vi "1_Sin(x)_Cos(x)(Training).vi"() -> ()   [LabVIEW 2020]
uses:
  <vilib>/Ngene/DeepLTK/Toolkit/NN_Train/Controls/NN_Train_Params.ctl
  <vilib>/Ngene/DeepLTK/Toolkit/NN_Train/Controls/NN_Train_Optimizer.ctl
  <vilib>/Ngene/DeepLTK/Toolkit/NN_Train/Controls/NN_Train_Data_Sampling.ctl
  <vilib>/Ngene/DeepLTK/Toolkit/NN_Train/Controls/NN_LR_Policy_Cfg.ctl
  <vilib>/Ngene/DeepLTK/Toolkit/NN_Train/Controls/NN_LR_Policy_Type.ctl
  <vilib>/Ngene/DeepLTK/Toolkit/NN_Train/Controls/NN_Train_Session_Data.ctl
  <vilib>/Ngene/DeepLTK/Toolkit/NN_Layers/Layers/FC/Controls/NN_Layer_Config(FC).ctl
  <vilib>/Ngene/DeepLTK/Toolkit/NN_Activations/Controls/NN_Activation_Type.ctl
  <vilib>/Ngene/DeepLTK/Toolkit/NN_Layers/Controls/NN_Layer_Init_Params.ctl
  <vilib>/Ngene/DeepLTK/Toolkit/NN_Layers/Controls/NN_Layer_Weight_Init_Type.ctl
  <vilib>/Ngene/DeepLTK/Toolkit/NN_Network/Controls/NN_Save_Before_Destroy_Options.ctl
  <vilib>/Ngene/DeepLTK/Toolkit/NN_Network/Controls/NN_Device.ctl
  <vilib>/Ngene/DeepLTK/Toolkit/NN_Layers/Layers/Input/Controls/NN_Layer_Config(Input1D).ctl
  <vilib>/Ngene/DeepLTK/Toolkit/NN_Data/API/DataSet_Types/NN_DataSet(In1D_Out1D).ctl
  <vilib>/Ngene/DeepLTK/Toolkit/NN_Data/API/DataRef_Types/NN_Data_ref(2D_SGL).ctl
  <vilib>/Ngene/DeepLTK/Toolkit/NN_Data/API/DataRef_Types/NN_Data_ref(1D_I32).ctl
  <vilib>/Analysis/1siggen.llb/Ramp Pattern by Samples.vi
  <vilib>/Ngene/DeepLTK/Toolkit/NN_Layers/Layers/Input/NN_Layer_Create(Input1D).vi
  <vilib>/Ngene/DeepLTK/Toolkit/NN_Layers/Layers/FC/NN_Layer_Create(FC).vi
  <vilib>/Ngene/DeepLTK/Toolkit/NN_Train/Loss_Functions/NN_Set_Loss(MSE).vi
  <vilib>/Ngene/DeepLTK/Toolkit/NN_Train/SubVIs/Dataset_Checks/NN_Check_Dataset(In1D_Out1D).vi
  <vilib>/Ngene/DeepLTK/Toolkit/NN_Data/subVIs/Get_Data_Vals/NN_Data_Get_ValByRef(2D_SGL).vi
  <vilib>/Ngene/DeepLTK/Toolkit/NN_Network/subVIs/NN_Predict/NN_Predict(In1D_Out1D).vi
  <vilib>/Ngene/DeepLTK/Toolkit/NN_Train/Eval_Loss/NN_Eval_Test_Error_Loss/NN_Eval(In1D_Out1D).vi
  <vilib>/Ngene/DeepLTK/Toolkit/Deep_Learning_Toolkit_by_Ngene.lvlib
  <vilib>/Analysis/NI_AALBase.lvlib
panel:
  out "Cos(x): Predictions vs Ground Truths":sgl[][](graph)
  out "Loop Time":dbl=0.043440699999337085 format="%#_4p"
  out "Test Loss":sgl=0.00088836974
  out "Training Loss":sgl=0.00065941934
  in  "Stop":bool
  out "Loss Graphs":cluster{"Loss":sgl, "Test Loss":sgl}(graph)={"Loss"=0.00065941934, "Test Loss"=0.0007708679}
  in  "# of Sine Cycles":dbl=5.0
  out "Sin(x): Predictions vs Ground Truths":sgl[][](graph)
  in  "Eval?":bool=TRUE
  out "Session Data":T1={"Epochs"=464.512, "Tot_Iter"=7258, "LR"=0.0025, "LR_iter"=7259}
  in  "LR_Decay_Params":T2={"Policy_Type"=enum."Step", "LR0"=0.01, "k"=200.0, "WarmUp_Policy"=enum."Ramp", "WarmUp_Iter"=100, "WarmUp_Ratio"=10.0} {"WarmUp_Ratio" min=1; "WarmUp_Iter" min=1; "LR0" format="%.7f"}
  in  "NN_Train_Params":T4={"Optimizer"=enum."Adam", "Beta_1"=0.9, "Beta_2"=0.999, "Weight Decay(L1)"=1e-08, "Weight Decay(L2)"=1e-08, "Data_Sampling"=enum."Random"}
  # "Overview: Demonstrates the usage of DeepLTK (Deep Learning Toolkit for LabVIEW) for solving a simple regression problem of modeling sin(x) and cos(x) function.\nRequirements: DeepLTK - Deep Learning Toolkit for LabVIEW (https://www.ngene.co/deep-learning-toolkit-for-labview)\nInstructions:\n1. Run the VI with default configurations.\n2. Observe how the training loss is decreasing.\n3. Periodically press \"Eval?\" button to observe \"Test Loss\" and performance of the model on Test Dataset\n4. Press \"Stop\" when \"Test Loss\" is is not decreasing. ~500 epochs\nMore Examples:  https://github.com/ngenehub/deepltk_examples"
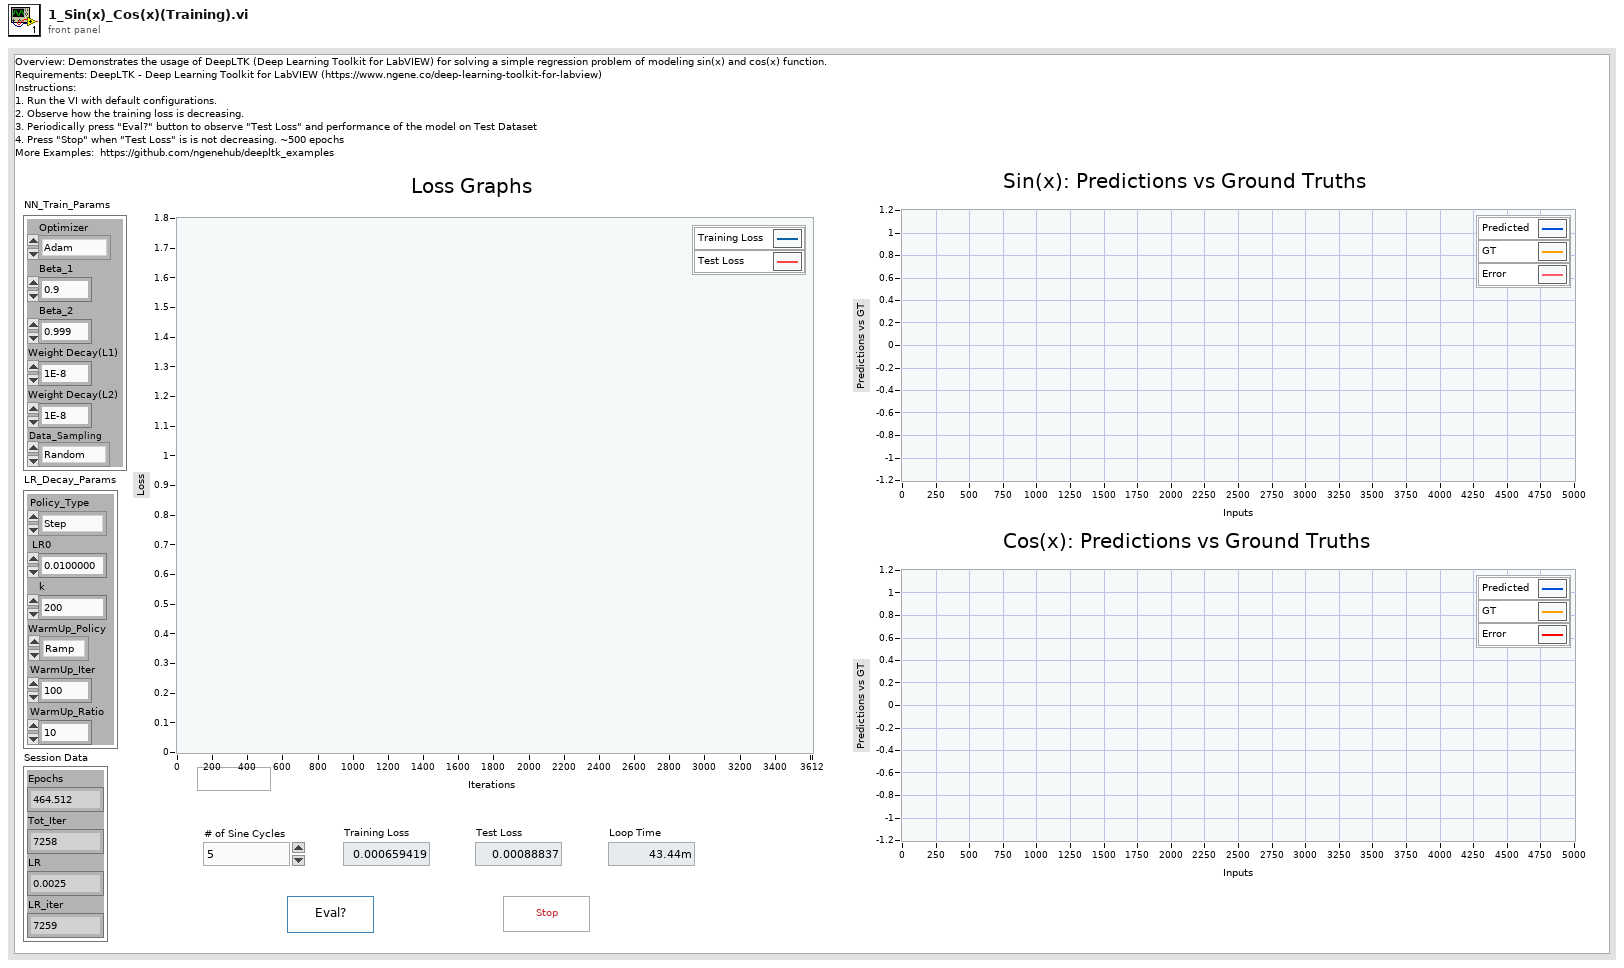
[diagram p1: front panel]
types:
  T1 = typedef "Deep_Learning_Toolkit_by_Ngene.lvlib/NN_Train_Session_Data.ctl" = cluster{"Epochs":sgl, "Tot_Iter":i32, "LR":sgl, "LR_iter":i32}
  T2 = typedef "Deep_Learning_Toolkit_by_Ngene.lvlib/NN_LR_Policy_Cfg.ctl" = cluster{"Policy_Type":T3, "LR0":dbl, "k":sgl, "WarmUp_Policy":enum16{"Step", "Ramp"}, "WarmUp_Iter":i32, "WarmUp_Ratio":sgl}
  T3 = typedef "Deep_Learning_Toolkit_by_Ngene.lvlib/NN_LR_Policy_Type.ctl" = enum16{"Manual", "Step", "Exp", "1/t"}
  T4 = typedef "Deep_Learning_Toolkit_by_Ngene.lvlib/NN_Train_Params.ctl" = cluster{"Optimizer":T5, "Beta_1":sgl, "Beta_2":sgl, "Weight Decay(L1)":sgl, "Weight Decay(L2)":sgl, "Data_Sampling":T6}
  T5 = typedef "Deep_Learning_Toolkit_by_Ngene.lvlib/NN_Train_Optimizer.ctl" = enum16{"SGD", "Adam", "Adagrad", "Adadelta", "RMSProp", "Nesterov"}
  T6 = typedef "Deep_Learning_Toolkit_by_Ngene.lvlib/NN_Train_Data_Sampling.ctl" = enum16{"Random", "Sequential"}
  T7 = typedef "Deep_Learning_Toolkit_by_Ngene.lvlib/NN_DataSet(In1D_Out1D).ctl" = cluster{"Inputs Ref.":T8, "Outputs Ref.":T8, "Dims_In":i32, "Dataset_Size":i32, "Outputs_idx Ref.":T9, "Dims_Out":i32, "Labels":string[], "File Paths":path[]}
  T8 = typedef "Deep_Learning_Toolkit_by_Ngene.lvlib/NN_Data_ref(2D_SGL).ctl" = refnum<data-value>
  T9 = typedef "Deep_Learning_Toolkit_by_Ngene.lvlib/NN_Data_ref(1D_I32).ctl" = refnum<data-value>
  T10 = typedef "Deep_Learning_Toolkit_by_Ngene.lvlib/NN_Layer_Config(Input1D).ctl" = cluster{"Name":string, "Size":i32}
  T11 = typedef "Deep_Learning_Toolkit_by_Ngene.lvlib/NN_Device.ctl" = enum16{"CPU", "GPU"}
  T12 = typedef "Deep_Learning_Toolkit_by_Ngene.lvlib/NN_Save_Before_Destroy_Options.ctl" = cluster{"CFG?":bool, "Weights?":bool, "Render?":bool}
  T13 = typedef "Deep_Learning_Toolkit_by_Ngene.lvlib/NN_Layer_Config(FC).ctl" = cluster{"Name":string, "Size":i32, "BN":bool, "Activation":T14, "Init_Params":T15, "Custom_Params":string}
  T14 = typedef "Deep_Learning_Toolkit_by_Ngene.lvlib/NN_Activation_Type.ctl" = enum16{"Sigmoid", "ReLU", "LReLU", "ReLU6", "tanh", "Swish", "Mish", "None"}
  T15 = typedef "Deep_Learning_Toolkit_by_Ngene.lvlib/NN_Layer_Init_Params.ctl" = cluster{"Init_Type":T16, "Value":sgl}
  T16 = typedef "Deep_Learning_Toolkit_by_Ngene.lvlib/NN_Layer_Weight_Init_Type.ctl" = enum16{"Const", "Uniform", "Gaussian", "Xavier"}
  T17 = typedef "Deep_Learning_Toolkit_by_Ngene.lvlib/NN.ctl" = cluster{"Name":string, "No of Layers":i32, "mBatch":i32, "Layers":T18[], "Dimty":T19, "Dims_In":T20, "Dims_Out":T20, "Working_Dir":path, "Train?":bool, "Train_Params":T4, "LR_Update_Policy":T2, "Session Data":T1, "Ground_truth":T21, "NNg_hdls":T22, "NN_Device":T11, "GPU Id":i32, "Labels":string[], "Receptive Field":T23[], "Loss_Type":T24, "Loss_Cfg_Prms":variant}
  T18 = typedef "Deep_Learning_Toolkit_by_Ngene.lvlib/NN_Layer_ref.ctl" = refnum<data-value>
  T19 = typedef "Deep_Learning_Toolkit_by_Ngene.lvlib/NN_In_Out_Dim-ty.ctl" = enum8{"In1D_Out1D", "In3D_Out1D", "In3D_Out3D", "In3D_OutBBox"}
  T20 = typedef "Deep_Learning_Toolkit_by_Ngene.lvlib/NN_Dims(C,H,W).ctl" = cluster{"C":i32, "H":i32, "W":i32}
  T21 = typedef "Deep_Learning_Toolkit_by_Ngene.lvlib/NN_Ground_truth.ctl" = cluster{"Y":variant, "Y_idx":T9}
  T22 = typedef "Deep_Learning_Toolkit_by_Ngene.lvlib/nng_cuda_handles.ctl" = cluster{"cudnn":u64, "cublas":u64, "stream":u64, "curand":u64}
  T23 = typedef "Deep_Learning_Toolkit_by_Ngene.lvlib/NN_Dims(V,H).ctl" = cluster{"V":i32, "H":i32}
  T24 = typedef "Deep_Learning_Toolkit_by_Ngene.lvlib/NN_Loss_Type.ctl" = enum16{"None", "MSE", "CrossEntropy", "YOLO_v2"}
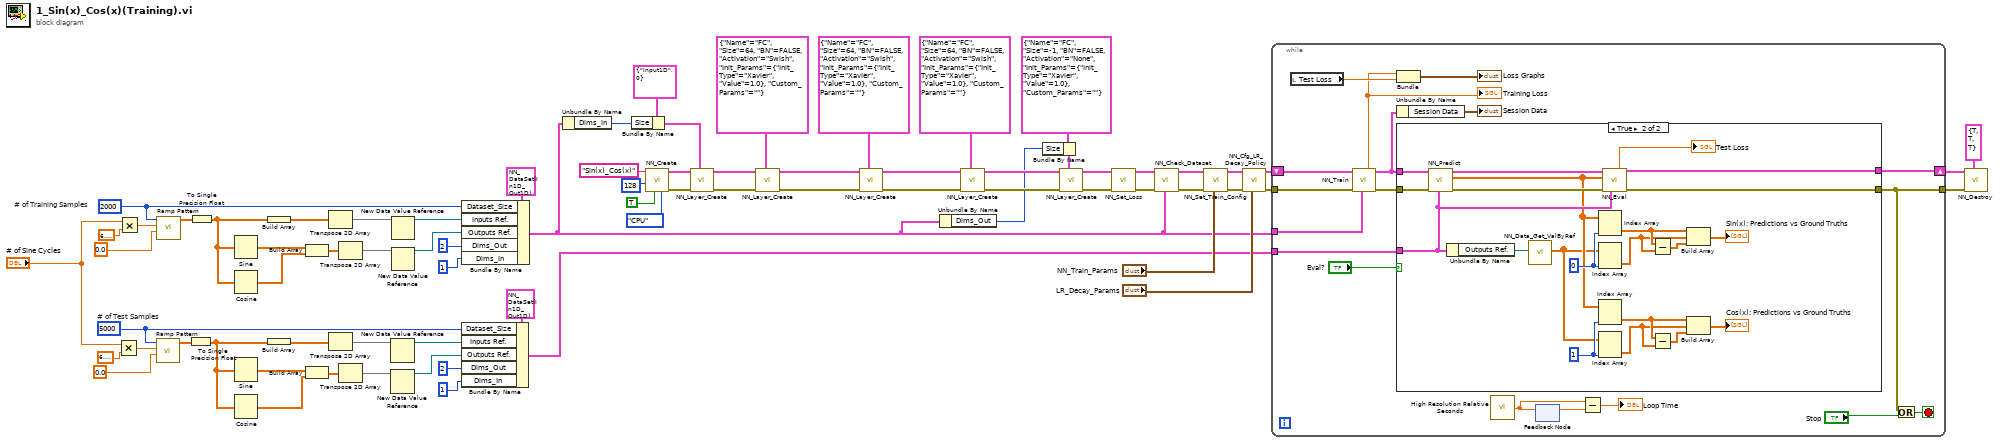
[diagram p0: block diagram]
diagram:
  w66 = 2000  # # of Training Samples
  w71 = 5000  # # of Test Samples
  n1 = Multiply(x="# of Sine Cycles", y=6.283185307179586) -> (x*y=w74:dbl)
  n2 = Multiply(x="# of Sine Cycles", y=6.283185307179586) -> (x*y=w69:dbl)
  n3 = call-poly <vilib>:"Ramp Pattern.vi"("start"=0.0, "end"=w74, "samples"=w71) -> ("Ramp Pattern"=w73:dbl[])  [unwired: 7 in, 1 out]
  n4 = call-poly <vilib>:"Ramp Pattern.vi"("start"=0.0, "end"=w69, "samples"=w66) -> ("Ramp Pattern"=w68:dbl[])  [unwired: 7 in, 1 out]
  n5 = To Single Precision Float(number=w73) -> (single precision float=w64:sgl[])
  n6 = To Single Precision Float(number=w68) -> (single precision float=w57:sgl[])
  n7 = Sine(x=w57) -> (sin(x)=w59:sgl[])
  n8 = Cosine(x=w57) -> (cos(x)=w58:sgl[])
  n9 = Sine(x=w64) -> (sin(x)=w61:sgl[])
  n10 = Cosine(x=w64) -> (cos(x)=w62:sgl[])
  n11 = Build Array(w57) -> (w53:sgl[][])
  n12 = Build Array(w64) -> (w55:sgl[][])
  n13 = Build Array(w59, w58) -> (w60:sgl[][])
  n14 = Build Array(w61, w62) -> (w63:sgl[][])
  n15 = Transpose 2D Array(2D array=w53) -> (transposed array=w2:sgl[][])
  n16 = Transpose 2D Array(2D array=w55) -> (transposed array=w1:sgl[][])
  n17 = Transpose 2D Array(2D array=w60) -> (transposed array=w56:sgl[][])
  n18 = Transpose 2D Array(2D array=w63) -> (transposed array=w54:sgl[][])
  n19 = New Data Value Reference(data value=w1) -> (data value reference=w21:refnum<data-value>)  [unwired: 1 in, 1 out]
  n20 = New Data Value Reference(data value=w54) -> (data value reference=w20:refnum<data-value>)  [unwired: 1 in, 1 out]
  n21 = New Data Value Reference(data value=w2) -> (data value reference=w17:refnum<data-value>)  [unwired: 1 in, 1 out]
  n22 = New Data Value Reference(data value=w56) -> (data value reference=w16:refnum<data-value>)  [unwired: 1 in, 1 out]
  n23 = Bundle By Name(cluster=T7 {"Inputs Ref."=refnum, "Outputs Ref."=refnum, "Dims_In"=0, "Dataset_Size"=0, "Outputs_idx Ref."=refnum, "Dims_Out"=0, "Labels"=[], "File Paths"=[]} ("Dataset(In1D_Out1D)"), "Dataset_Size"=w71, "Inputs Ref."=w21, "Outputs Ref."=w20, "Dims_Out"=2, "Dims_In"=1 ("Dims_Out")) -> (w19:T7)
  n24 = Bundle By Name(cluster=T7 {"Inputs Ref."=refnum, "Outputs Ref."=refnum, "Dims_In"=0, "Dataset_Size"=0, "Outputs_idx Ref."=refnum, "Dims_Out"=0, "Labels"=[], "File Paths"=[]} ("Dataset(In1D_Out1D)"), "Dataset_Size"=w66, "Inputs Ref."=w17, "Outputs Ref."=w16, "Dims_Out"=2, "Dims_In"=1 ("Dims_Out")) -> (w6:T7)
  n25 = Unbundle By Name(w6) -> ("Dims_In"=w26:i32)
  n26 = Bundle By Name(cluster=T10 {"Name"="Input1D", "Size"=0} ("Input1D_Cfg"), "Size"=w26) -> (w44:T10)
  n27 = call <vilib>:"NN_Create.vi"("NN_Device"=NN_Device."CPU", "Train? (false)"=TRUE, "mBatch (1)"=128, "Name"="Sin(x)_Cos(x)") -> ("error out"=w49:errorcluster, "NN out"=w50:T17)  [unwired: 6 in]
  n28 = call-poly <vilib>:"NN_Layer_Create.vi"("Input1D_Cfg"=w44, "error in (no error)"=w49, "NN in"=w50) -> ("error out"=w52:errorcluster, "NN out"=w51:T17)  [unwired: 6 in, 1 out]
  n29 = call-poly <vilib>:"NN_Layer_Create.vi"("FC_Cfg"=T13 {"Name"="FC", "Size"=64, "BN"=FALSE, "Activation"=enum."Swish", "Init_Params"={"Init_Type"=enum."Xavier", "Value"=1.0}, "Custom_Params"=""}, "error in (no error)"=w52, "NN in"=w51) -> ("error out"=w24:errorcluster, "NN out"=w25:T17)  [unwired: 6 in, 1 out]
  n30 = call-poly <vilib>:"NN_Layer_Create.vi"("FC_Cfg"=T13 {"Name"="FC", "Size"=64, "BN"=FALSE, "Activation"=enum."Swish", "Init_Params"={"Init_Type"=enum."Xavier", "Value"=1.0}, "Custom_Params"=""}, "error in (no error)"=w24, "NN in"=w25) -> ("error out"=w12:errorcluster, "NN out"=w13:T17)  [unwired: 6 in, 1 out]
  n31 = Unbundle By Name(w6) -> ("Dims_Out"=w5:i32)
  n32 = call-poly <vilib>:"NN_Layer_Create.vi"("FC_Cfg"=T13 {"Name"="FC", "Size"=64, "BN"=FALSE, "Activation"=enum."Swish", "Init_Params"={"Init_Type"=enum."Xavier", "Value"=1.0}, "Custom_Params"=""}, "error in (no error)"=w12, "NN in"=w13) -> ("error out"=w10:errorcluster, "NN out"=w11:T17)  [unwired: 6 in, 1 out]
  n33 = Bundle By Name(cluster=T13 {"Name"="FC", "Size"=-1, "BN"=FALSE, "Activation"=enum."None", "Init_Params"={"Init_Type"=enum."Xavier", "Value"=1.0}, "Custom_Params"=""} ("FC_Cfg"), "Size"=w5) -> (w3:T13)
  n34 = call-poly <vilib>:"NN_Layer_Create.vi"("FC_Cfg"=w3, "error in (no error)"=w10, "NN in"=w11) -> ("error out"=w28:errorcluster, "NN out"=w27:T17)  [unwired: 6 in, 1 out]
  n35 = call-poly <vilib>:"NN_Set_Loss.vi"("error in (no error)"=w28, "NN in"=w27) -> ("error out"=w30:errorcluster, "NN out"=w42:T17)  [unwired: 8 in]
  n36 = call-poly <vilib>:"NN_Check_Dataset.vi"("Dataset"=w6, "error in (no error)"=w30, "NN in"=w42) -> ("error out"=w29:errorcluster, "NN out"=w31:T17)  [unwired: 7 in]
  n37 = call <vilib>:"NN_Set_Train_Config.vi"("NN_Train_Params"="NN_Train_Params", "error in (no error)"=w29, "NN in"=w31) -> ("error out"=w36:errorcluster, "NN out"=w41:T17)  [unwired: 7 in]
  n38 = call <vilib>:"NN_Cfg_LR_Decay_Policy.vi"("LR_Decay_Params"="LR_Decay_Params", "error in (no error)"=w36, "NN in"=w41) -> ("error out"=w35:errorcluster, "NN out"=w37:T17)  [unwired: 7 in]
  n39 = while {
    tunnel: w35 -> [w92]
    tunnel: w6 -> [w84]
    shift-right: [w88] -> w39
    shift-left: w37 -> [w93]
    tunnel: [w83] -> w38
    tunnel: w19 -> [w82]
    stop <- w91 stop-if-true
    n40 = local read "Test Loss"() -> (w85:sgl)
    n41 = call <vilib>:"NN_Train.vi"("Train Dataset"=w84, "error in (no error)"=w92, "NN in"=w93) -> ("error out"=w87:errorcluster, "NN out"=w90:T17, "Loss"=w76:sgl)  [unwired: 5 in, 1 out]
    "Training Loss" <- w76
    n42 = Bundle("Loss"=w76, "Test Loss"=w85) -> (→"Loss Graphs":cluster{"Loss":sgl, "Test Loss":sgl})  [unwired: 1 in]
    n43 = Unbundle By Name(w90) -> ("Session Data"=→"Session Data":T1)
    n44 = case shown="True" "Eval?" {
      tunnel: w90 -> [w95 w112]
      tunnel: [w95 w116] -> w88
      tunnel: w87 -> [w94 w111]
      tunnel: [w94 w115] -> w83
      tunnel: w82 -> [_ w110]
      frame False {
      }
      frame True {
        w106 = 1 ("disabled index (col)")
        w108 = 0 ("disabled index (col)")
        n45 = call-poly <vilib>:"NN_Predict.vi"("Dataset"=w110, "error in (no error)"=w111, "NN in"=w112) -> ("error out"=w113:errorcluster, "Predictions"=w105:sgl[][], "NN out"=w114:T17)  [unwired: 6 in]
        n46 = Unbundle By Name(w110) -> ("Outputs Ref."=w109:T8)
        n47 = call-poly <vilib>:"NN_Data_Get_ValByRef.vi"("DVR(2D_SGL)"=w109) -> ("Value(2D_SGL)"=w104:sgl[][])  [unwired: 7 in, 1 out]
        n48 = Index Array(array=w105, index (col)=w108) -> (element=w101:sgl[])  [unwired: 1 in]
        n49 = Index Array(array=w104, index (col)=w108) -> (element=w99:sgl[])  [unwired: 1 in]
        n50 = Index Array(array=w105, index (col)=w106) -> (element=w97:sgl[])  [unwired: 1 in]
        n51 = Index Array(array=w104, index (col)=w106) -> (element=w96:sgl[])  [unwired: 1 in]
        n52 = call-poly <vilib>:"NN_Eval.vi"("NN in"=w114, "Predictions"=w105, "error in (no error)"=w113, "Dataset"=w110) -> ("Loss"=→"Test Loss":sgl, "NN out"=w116:T17, "error out"=w115:errorcluster)  [unwired: 7 in, 2 out]
        n53 = Subtract(x=w101, y=w99) -> (x-y=w100:sgl[])
        n54 = Subtract(x=w97, y=w96) -> (x-y=w98:sgl[])
        n55 = Build Array(w101, w99, w100) -> (→"Sin(x): Predictions vs Ground Truths":sgl[][])
        n56 = Build Array(w97, w96, w98) -> (→"Cos(x): Predictions vs Ground Truths":sgl[][])
      }
    }
    n57 = call <vilib>:"High Resolution Relative Seconds.vi"() -> ("relative seconds"=w81:dbl)
    n58 = feedback-in #1(w81) -> ()
    n59 = feedback #1() -> (w80:dbl)  [unwired: 1 in]
    n60 = Subtract(x=w81, y=w80) -> (x-y=→"Loop Time":dbl)
    n61 = Or(x=w83, y="Stop") -> (x .or. y?=w91:bool)
  }
  n62 = call <vilib>:"NN_Destroy.vi"("Save (T, T, T)"=T12 {"CFG?"=TRUE, "Weights?"=TRUE, "Render?"=TRUE}, "error in (no error)"=w38, "NN in"=w39) -> ()  [unwired: 8 in, 1 out]
